vi "Create_Trajectory_Build_Trajectory_Field_Plot.vi"(9 "TrackWidth_Meters":dbl, 10 "WayPoints":T1[](array[typedef]) {"WEIGHT" format="%13.3f"; "ANGLE" format="%13.3f"; "Y" format="%13.3f"; "X" format="%13.3f"}, 11 "States":T2[](array[typedef]) {"POSE"."ROTATION"."SIN" format="%13.4f"; "POSE"."ROTATION"."COS" format="%13.4f"; "POSE"."ROTATION"."VALUE" format="%13.4f"; "POSE"."TRANSLATION"."Y" format="%14.3f"; "POSE"."TRANSLATION"."X" format="%14.3f"}) -> (3 "Array":cluster{dbl[], dbl[]}[](array[cluster]))   [LabVIEW 2019]
uses:
  <vilib>/Rock Robotics/WPI/ThirdParty/JAS_Junk/TrajLib/TRAJ_STATE.ctl
  <vilib>/Rock Robotics/WPI/ThirdParty/JAS_Junk/TrajLib/POSE2D.ctl
  <vilib>/Rock Robotics/WPI/ThirdParty/JAS_Junk/TrajLib/TRANSLATION2D.ctl
  <vilib>/Rock Robotics/WPI/ThirdParty/JAS_Junk/TrajLib/ROTATION2D.ctl
  <vilib>/Rock Robotics/WPI/ThirdParty/JAS_Junk/TrajLib/DISPLAY_WEIGHTED_WAYPOINT.ctl
  <vilib>/Rock Robotics/WPI/ThirdParty/JAS_Junk/TrajLib/Trajectory_Library.lvlib
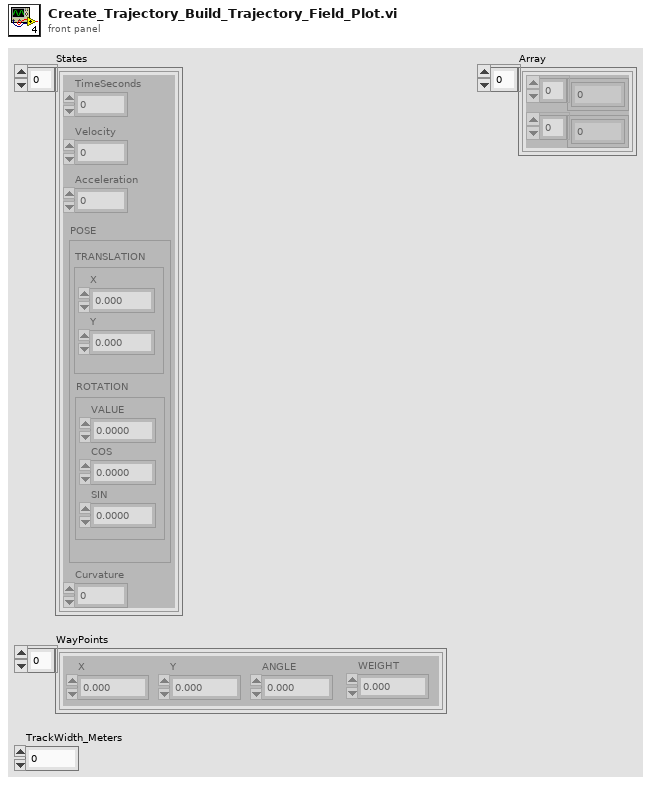
[diagram p1: front panel]
types:
  T1 = typedef "Trajectory_Library.lvlib/DISPLAY_WEIGHTED_WAYPOINT.ctl" = cluster{"X":dbl, "Y":dbl, "ANGLE":dbl, "WEIGHT":dbl}
  T2 = typedef "Trajectory_Library.lvlib/TRAJ_STATE.ctl" = cluster{"TimeSeconds":dbl, "Velocity":dbl, "Acceleration":dbl, "POSE":T3, "Curvature":dbl}
  T3 = typedef "Trajectory_Library.lvlib/POSE2D.ctl" = cluster{"TRANSLATION":T4, "ROTATION":T5}
  T4 = typedef "Trajectory_Library.lvlib/TRANSLATION2D.ctl" = cluster{"X":dbl, "Y":dbl}
  T5 = typedef "Trajectory_Library.lvlib/ROTATION2D.ctl" = cluster{"VALUE":dbl, "COS":dbl, "SIN":dbl}
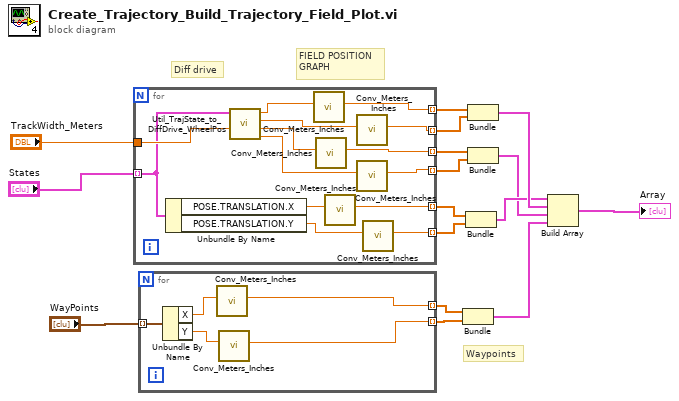
[diagram p0: block diagram]
diagram:
  # "Waypoints"
  # "Diff drive"
  # "FIELD POSITION\nGRAPH"
  n1 = for {
    tunnel: "States" -> [w21] mode=indexing
    tunnel: "TrackWidth_Meters" -> [w30]
    tunnel: [w28] -> w2 mode=indexing
    tunnel: [w27] -> w3 mode=indexing
    tunnel: [w24] -> w4 mode=indexing
    tunnel: [w22] -> w5 mode=indexing
    tunnel: [w18] -> w9 mode=indexing
    tunnel: [w17] -> w10 mode=indexing
    n2 = Unbundle By Name(w21) -> ("POSE.TRANSLATION.X"=w20:dbl, "POSE.TRANSLATION.Y"=w19:dbl)
    n3 = call <vilib>:"Util_TrajState_to_DiffDrive_WheelPos.vi"("Wheelbase"=w30, "TRAJ_STATE"=w21) -> ("Right Y"=w23:dbl, "Right X"=w25:dbl, "Left Y"=w26:dbl, "Left X"=w29:dbl)  [unwired: 6 in]
    n4 = call <vilib>:"Conv_Meters_Inches.vi"("Meters"=w29) -> ("Inches"=w28:dbl)  [unwired: 10 in]
    n5 = call <vilib>:"Conv_Meters_Inches.vi"("Meters"=w25) -> ("Inches"=w24:dbl)  [unwired: 10 in]
    n6 = call <vilib>:"Conv_Meters_Inches.vi"("Meters"=w20) -> ("Inches"=w17:dbl)  [unwired: 10 in]
    n7 = call <vilib>:"Conv_Meters_Inches.vi"("Meters"=w26) -> ("Inches"=w27:dbl)  [unwired: 10 in]
    n8 = call <vilib>:"Conv_Meters_Inches.vi"("Meters"=w23) -> ("Inches"=w22:dbl)  [unwired: 10 in]
    n9 = call <vilib>:"Conv_Meters_Inches.vi"("Meters"=w19) -> ("Inches"=w18:dbl)  [unwired: 10 in]
  }
  n10 = for {
    tunnel: "WayPoints" -> [w35] mode=indexing
    tunnel: [w32] -> w13 mode=indexing
    tunnel: [w31] -> w14 mode=indexing
    n11 = Unbundle By Name(w35) -> ("X"=w34:dbl, "Y"=w33:dbl)
    n12 = call <vilib>:"Conv_Meters_Inches.vi"("Meters"=w34) -> ("Inches"=w32:dbl)  [unwired: 10 in]
    n13 = call <vilib>:"Conv_Meters_Inches.vi"("Meters"=w33) -> ("Inches"=w31:dbl)  [unwired: 10 in]
  }
  n14 = Bundle(w13, w14) -> (w15:cluster{dbl[], dbl[]})  [unwired: 1 in]
  n15 = Bundle(w10, w9) -> (w7:cluster{dbl[], dbl[]})  [unwired: 1 in]
  n16 = Bundle(w2, w3) -> (w8:cluster{dbl[], dbl[]})  [unwired: 1 in]
  n17 = Bundle(w4, w5) -> (w6:cluster{dbl[], dbl[]})  [unwired: 1 in]
  n18 = Build Array(w7, w8, w6, w15) -> (→"Array":cluster{dbl[], dbl[]}[])
